vi "StabilizationSettings.vi"() -> ()   [LabVIEW 2012]
panel:
  in  "StabilizationSettings":T1
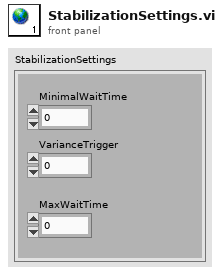
[diagram p1: front panel]
types:
  T1 = cluster{"MinimalWaitTime":u32, "VarianceTrigger":dbl, "MaxWaitTime":u32}
diagram:
